vi "FFTtoR,Theta.VI"   [LabVIEW 2020]
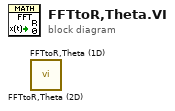
[diagram p0: block diagram]
diagram:
  n1 = call "FFTtoR,Theta (2D).VI"() -> ()  [unwired: 2 in, 2 out]
  n2 = call "FFTtoR,Theta (1D).VI"() -> ()  [unwired: 2 in, 2 out]
